vi "Voltage - Temp Conversion.vi"(11 "mean":dbl) -> (3 "Numeric":dbl)   [LabVIEW 2018]
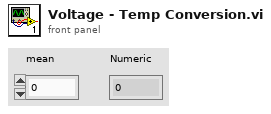
[diagram p1: front panel]
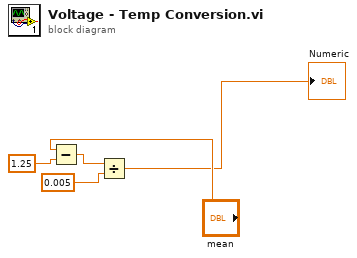
[diagram p0: block diagram]
diagram:
  n1 = Subtract(x="mean", y=1.25 ("minimum value")) -> (x-y=w1:dbl)
  n2 = Divide(x=w1, y=0.005 ("minimum value")) -> (x/y=→"Numeric":dbl)
